vi "探头窗口-16-服务器版.vi"() -> ()   [LabVIEW 2013]
panel:
  in  "外部停止命令？":bool=TRUE
  out "引用-探头属性[]":refnum<vi>
  out "引用-监测模式？":refnum<vi>
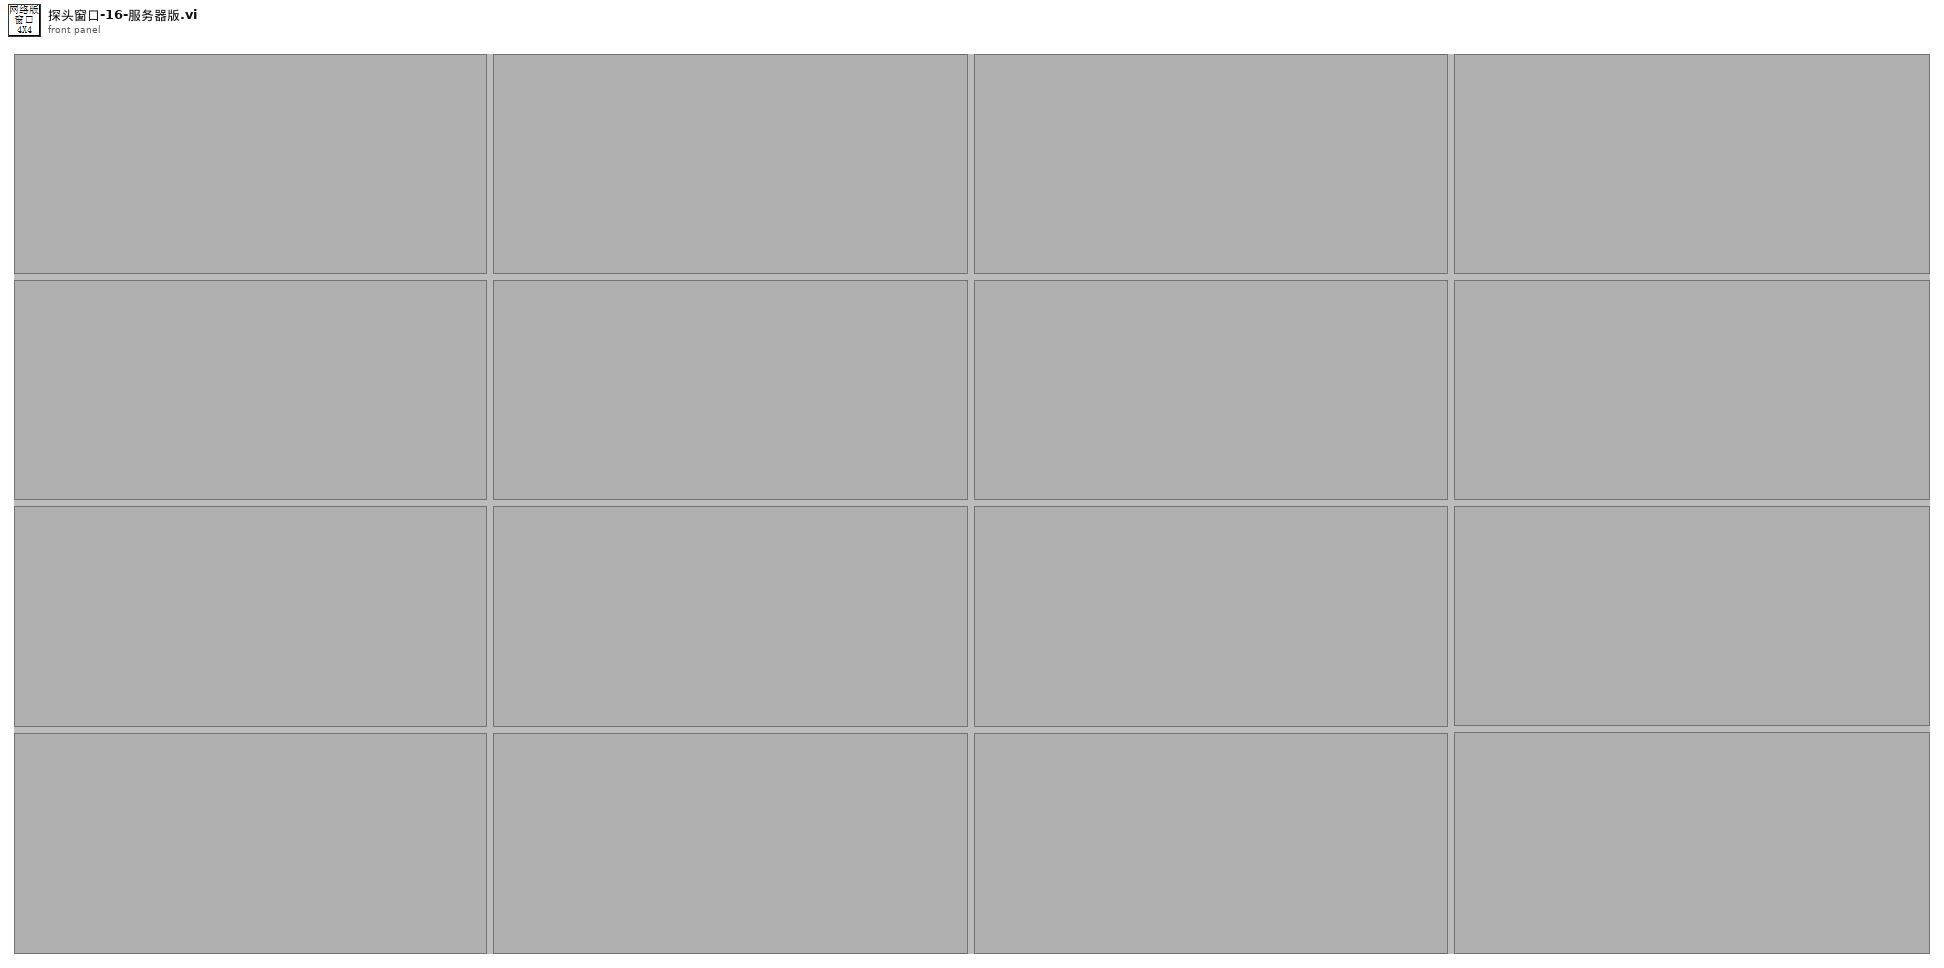
[diagram p1: front panel]
types:
  T1 = typedef "eventvkey.ctl" = enum16{"ASCII", "Enter", "Return", "Shift", "Ctrl", "Alt", "Cmd", "Opt", "Caps", "NumLock", "Clear", "Break", "Up", "Down", "Left", "Right", "Insert", "Delete", "Home", "End", "PageUp", "PageDown", "Escape", "Help", "Pause", "ScrollLock", "F1", "F2", "F3", "F4", "F5", "F6", "F7", "F8", "F9", "F10", "F11", "F12", "F13", "F14", "F15", "F16", "F17", "F18", "F19", "F20", "F21", "F22", "F23", "F24", "Play", "VolumeUp", "VolumeDown", "Mute", "Two Byte Char"}
  T2 = cluster{"探头地址与信息":cluster{"网络地址":cluster{"IP":string, "port":u16}, "探头信息":string}, "测量值":cluster{"时间":timestamp, "数值":dbl}, "限值":cluster{"限值1":dbl, "限值2":dbl}, "探头状态":enum16{"正常", "离线", "禁用", "一级报警", "二级报警"}}[]
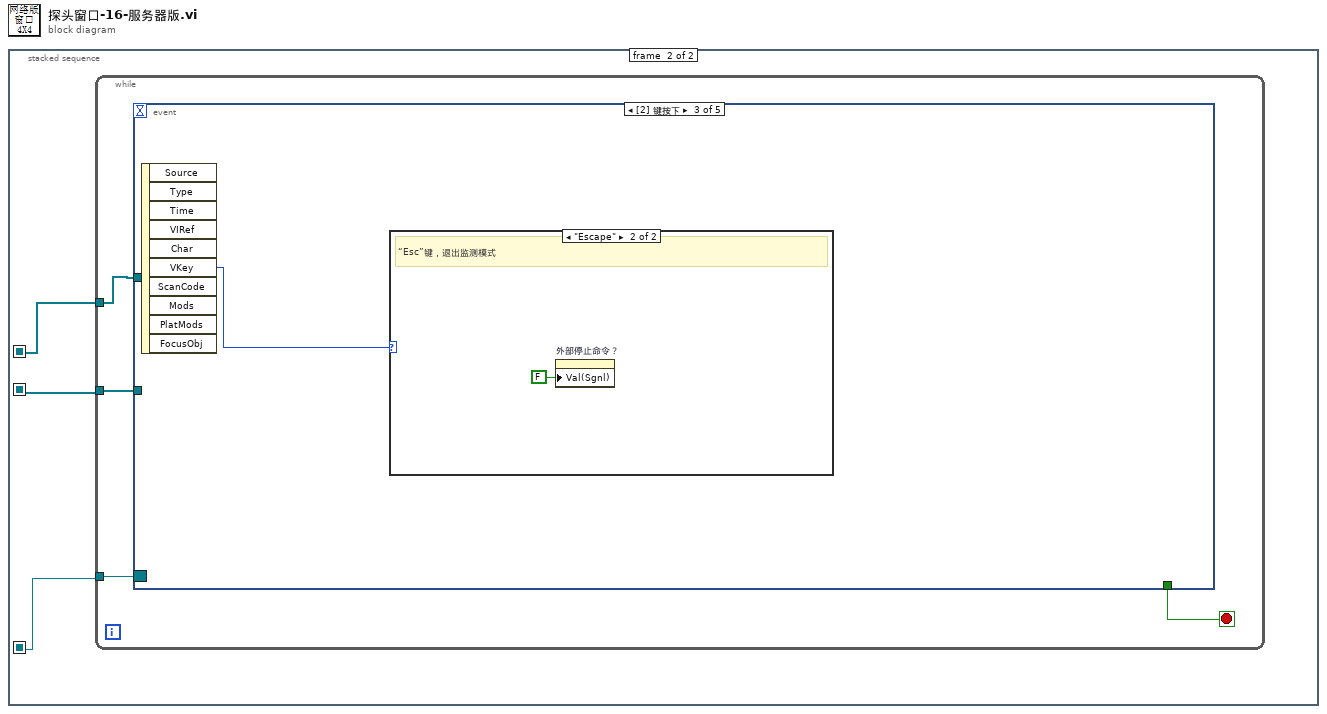
[diagram p0: block diagram]
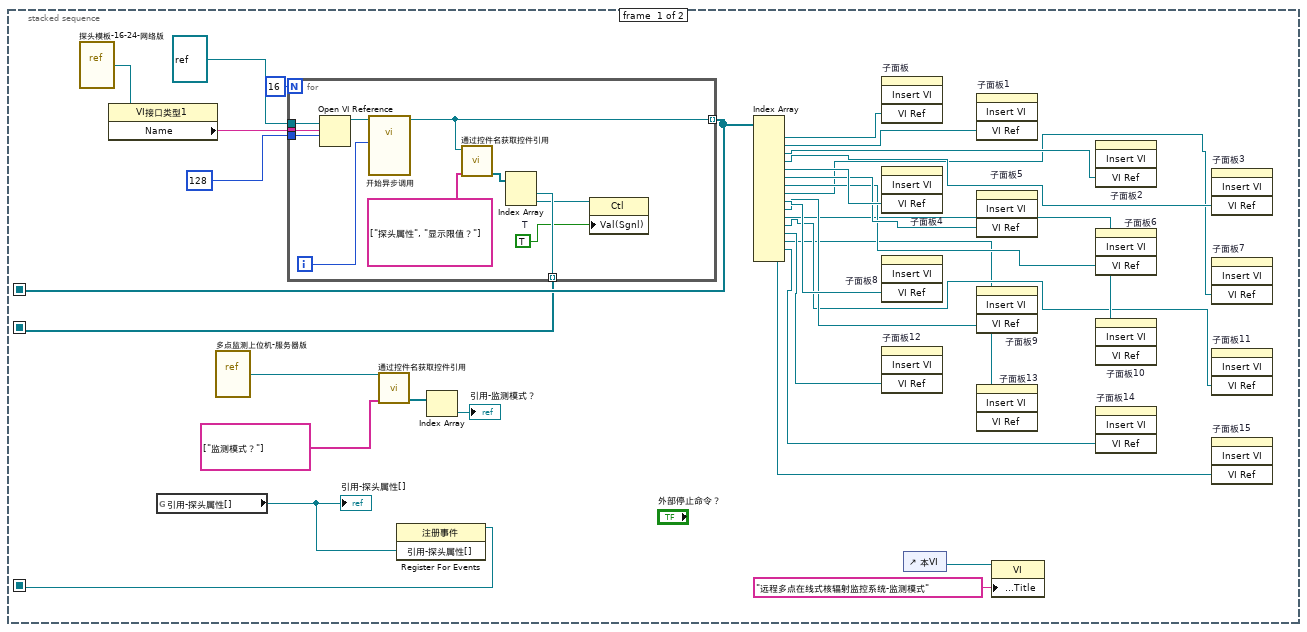
[diagram p2: hidden frame]
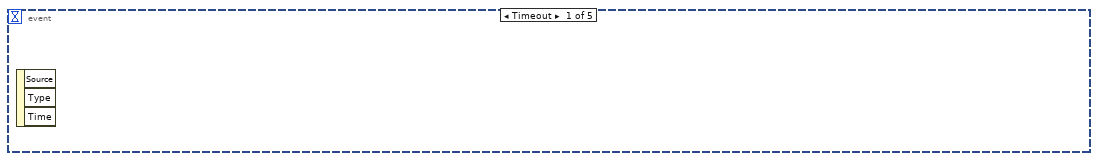
[diagram p3: hidden frame]
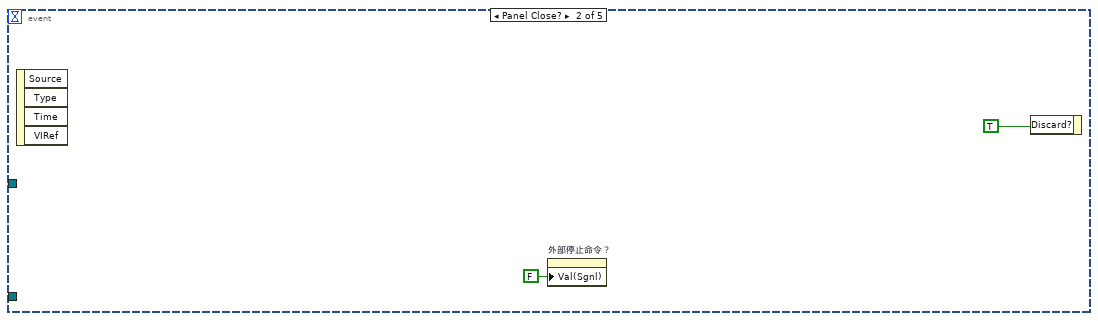
[diagram p4: hidden frame]
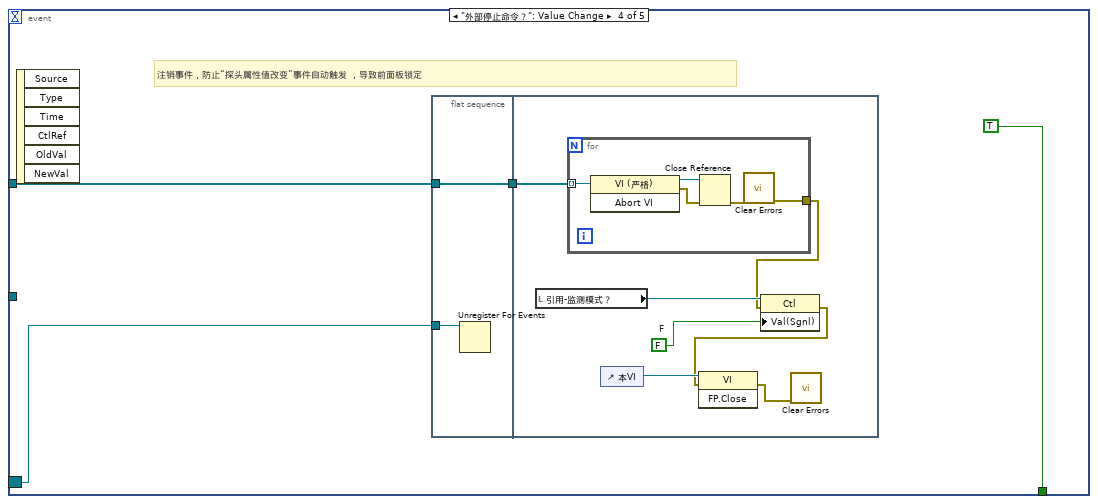
[diagram p6: hidden frame]
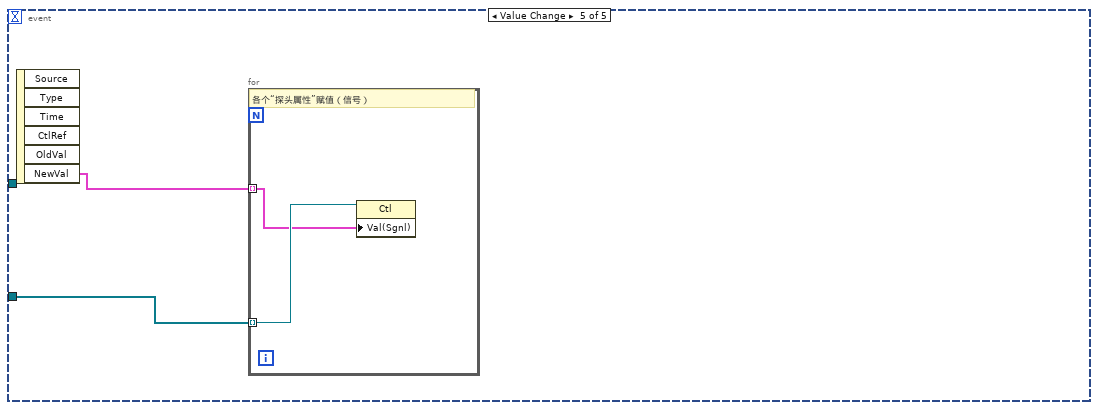
[diagram p7: hidden frame]
diagram:
  n1 = stacked-sequence {
    seq-local: [w26 _] -> [_ w45]
    seq-local: [w5 _] -> [_ w44]
    seq-local: [w3 _] -> [_ w43]
    frame #0 {
      n2 = vi-ref "探头模板-16-24-网络版.vi"() -> (w31:refnum<vi>)
      n3 = property class="VI接口类型1"(reference=w31) -> ("Name"=w30:string)  [unwired: 1 in, 2 out]
      n4 = global read "全局变量-35点监测.vi" "引用-探头属性[]"() -> (w4:refnum<vi>)
      "引用-探头属性[]" <- w4
      n5 = vi-ref "多点监测上位机-服务器版.vi"() -> (w6:refnum<vi>)
      n6 = for "For循环" {
        N: 16 -> [_]
        tunnel: w30 -> [w42]
        tunnel: 128 ("选项") -> [w41]
        tunnel: refnum<vi> refnum ("类型说明符VI引用句柄（仅用于类型）") -> [w40]
        tunnel: [w35] -> w26 mode=indexing
        tunnel: [w36] -> w5 mode=indexing
        i -> [w32]
        w33 = TRUE  # T
        n7 = Open VI Reference(type specifier VI Refnum (for type only)=w40, vi path=w42, options=w41) -> (vi reference=w37:refnum<vi>)  [unwired: 3 in, 1 out]
        n8 = call-by-ref "开始异步调用"(reference=w37, "探头序号"=w32) -> (reference out=w35:refnum<vi>)  [unwired: 12 in, 1 out]
        n9 = call "通过控件名获取控件引用.vi"("控件名数组"=string[] ["探头属性", "显示限值？"], "VI引用"=w35) -> ("控件引用输出"=w39:refnum<vi>[])  [unwired: 7 in, 2 out]
        n10 = Index Array(array=w39) -> (element #1=w36:refnum<vi>, element #2=w34:refnum<vi>)  [unwired: 2 in]
        n11 = property class="Ctl"(reference=w34, "Val(Sgnl)"=w33) -> ()  [unwired: 1 in, 2 out]
      }
      n12 = call "通过控件名获取控件引用.vi"("控件名数组"=string[] ["监测模式？"], "VI引用"=w6) -> ("控件引用输出"=w8:refnum<vi>[])  [unwired: 7 in, 2 out]
      n13 = register-events(w4) -> (reference out=w3:refnum<event-registration>)  [unwired: 2 in, 1 out]
      n14 = Index Array(array=w8) -> (element=→"引用-监测模式？":refnum<vi>)  [unwired: 1 in]
      n15 = Index Array(array=w26) -> (element #1=w25:refnum<vi>, element #2=w24:refnum<vi>, element #3=w23:refnum<vi>, element #4=w22:refnum<vi>, element #5=w21:refnum<vi>, element #6=w20:refnum<vi>, element #7=w19:refnum<vi>, element #8=w18:refnum<vi>, element #9=w17:refnum<vi>, element #10=w16:refnum<vi>, element #11=w15:refnum<vi>, element #12=w14:refnum<vi>, element #13=w13:refnum<vi>, element #14=w12:refnum<vi>, element #15=w11:refnum<vi>, element #16=w10:refnum<vi>)  [unwired: 16 in]
      n16 = invoke on="子面板" class="子面板" method="Insert VI"("VI Ref"=w25) -> ()  [unwired: 3 in, 4 out]
      n17 = invoke on="子面板4" class="SubPnl" method="Insert VI"("VI Ref"=w21) -> ()  [unwired: 3 in, 4 out]
      n18 = invoke on="子面板8" class="SubPnl" method="Insert VI"("VI Ref"=w17) -> ()  [unwired: 3 in, 4 out]
      n19 = invoke on="子面板12" class="SubPnl" method="Insert VI"("VI Ref"=w13) -> ()  [unwired: 3 in, 4 out]
      n20 = control-ref of="本VI"() -> (w2:refnum<vi>)
      n21 = invoke on="子面板1" class="SubPnl" method="Insert VI"("VI Ref"=w24) -> ()  [unwired: 3 in, 4 out]
      n22 = invoke on="子面板5" class="SubPnl" method="Insert VI"("VI Ref"=w20) -> ()  [unwired: 3 in, 4 out]
      n23 = invoke on="子面板9" class="SubPnl" method="Insert VI"("VI Ref"=w16) -> ()  [unwired: 3 in, 4 out]
      n24 = invoke on="子面板13" class="SubPnl" method="Insert VI"("VI Ref"=w12) -> ()  [unwired: 3 in, 4 out]
      n25 = property class="VI"(reference=w2, "Front Panel.Title"="远程多点在线式核辐射监控系统-监测模式" ("前面板窗口:标题")) -> ()  [unwired: 1 in, 2 out]
      n26 = invoke on="子面板2" class="SubPnl" method="Insert VI"("VI Ref"=w23) -> ()  [unwired: 3 in, 4 out]
      n27 = invoke on="子面板6" class="SubPnl" method="Insert VI"("VI Ref"=w19) -> ()  [unwired: 3 in, 4 out]
      n28 = invoke on="子面板10" class="SubPnl" method="Insert VI"("VI Ref"=w15) -> ()  [unwired: 3 in, 4 out]
      n29 = invoke on="子面板14" class="SubPnl" method="Insert VI"("VI Ref"=w11) -> ()  [unwired: 3 in, 4 out]
      n30 = invoke on="子面板3" class="SubPnl" method="Insert VI"("VI Ref"=w22) -> ()  [unwired: 3 in, 4 out]
      n31 = invoke on="子面板7" class="SubPnl" method="Insert VI"("VI Ref"=w18) -> ()  [unwired: 3 in, 4 out]
      n32 = invoke on="子面板11" class="SubPnl" method="Insert VI"("VI Ref"=w14) -> ()  [unwired: 3 in, 4 out]
      n33 = invoke on="子面板15" class="SubPnl" method="Insert VI"("VI Ref"=w10) -> ()  [unwired: 3 in, 4 out]
    }
    frame #1 {
      n34 = while {
        tunnel: w45 -> [w48]
        tunnel: w44 -> [w47]
        tunnel: w43 -> [w46]
        stop <- w49 stop-if-true
        n35 = event shown="[2] 键按下" {
          selector: w46 -> [_ _ _ w54 _]
          dyn-events: _ -> [_ _ _ _ _]
          timeout: _ -> [_ _ _ _ _]
          tunnel: [_ _ _ TRUE ("放弃？") _] -> w49
          tunnel: w48 -> [_ _ _ w56 _]
          tunnel: w47 -> [_ _ _ _ w72]
          event Timeout {
            n36 = event-data() -> ()  [unwired: 1 in, 3 out]
          }
          event Panel Close? {
            n37 = event-data() -> ()  [unwired: 1 in, 4 out]
            n38 = property on="外部停止命令？" class="Bool (严格)"("Val(Sgnl)"=FALSE ("值(信号)")) -> ()  [unwired: 2 in, 2 out]
            n39 = event-data("Discard?"=TRUE ("放弃？")) -> ()  [unwired: 1 in, 1 out]
          }
          event Key Down {
            n40 = event-data() -> ("VKey"=w52:T1)  [unwired: 1 in, 9 out]
            n41 = case shown="\"Escape\"" w52 {
              frame "ASCII", Default {
              }
              frame "Escape" {
                # "“Esc”键，退出监测模式"
                n42 = property on="外部停止命令？" class="Bool (严格)"("Val(Sgnl)"=FALSE ("值(信号)")) -> ()  [unwired: 2 in, 2 out]
              }
            }
          }
          event "外部停止命令？": Value Change {
            # "注销事件，防止“探头属性值改变”事件自动触发 ，导致前面板锁定"
            n43 = event-data() -> ()  [unwired: 1 in, 6 out]
            n44 = flat-sequence {
              tunnel: w56 -> [w59]
              tunnel: [w59] -> w55
              tunnel: w54 -> [w58]
              tunnel: w55 -> [w66]
              frame #0 {
                n45 = Unregister For Events(event registration refnum=w58) -> ()  [unwired: 1 in, 1 out]
              }
              frame #1 {
                w65 = FALSE  # F
                n46 = local read "引用-监测模式？"() -> (w64:refnum<vi>)
                n47 = for "For循环" {
                  tunnel: w66 -> [w71] mode=indexing
                  tunnel: [w67] -> w62
                  n48 = invoke class="VI (严格)" method="Abort VI"(reference=w71) -> (reference out=w69:refnum<vi>, error out=w70:errorcluster)  [unwired: 2 in, 1 out]
                  n49 = Close Reference(reference=w69, error in (no error)=w70) -> (error out=w68:errorcluster)
                  n50 = call <vilib>:"Clear Errors.vi"("error in (no error)"=w68) -> ("error out"=w67:errorcluster)  [unwired: 6 in]
                }
                n51 = control-ref of="本VI"() -> (w63:refnum<vi>)
                n52 = property class="Ctl"(reference=w64, error in=w62, "Val(Sgnl)"=w65) -> (error out=w61:errorcluster)  [unwired: 1 out]
                n53 = invoke class="VI" method="FP.Close"(reference=w63, error in=w61) -> (error out=w60:errorcluster)  [unwired: 1 in, 2 out]
                n54 = call <vilib>:"Clear Errors.vi"("error in (no error)"=w60) -> ()  [unwired: 6 in, 1 out]
              }
            }
          }
          event Value Change {
            n55 = event-data() -> ("NewVal"=w73:T2)  [unwired: 1 in, 5 out]
            n56 = for "For循环" {
              tunnel: w72 -> [w75] mode=indexing
              tunnel: w73 -> [w74] mode=indexing
              # "各个“探头属性”赋值（信号）"
              n57 = property class="Ctl"(reference=w75, "Val(Sgnl)"=w74) -> ()  [unwired: 1 in, 2 out]
            }
          }
        }
      }
    }
  }
